vi "IsValidFile.vi"(8 "error in (no error)":errorcluster, 11 "Source Path":path) -> (0 "error out":errorcluster, 2 "Valid File":bool, 3 "path out":path)   [LabVIEW 2023]
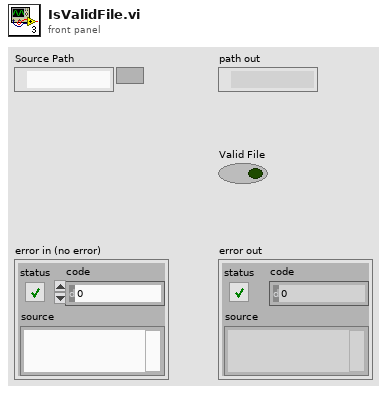
[diagram p1: front panel]
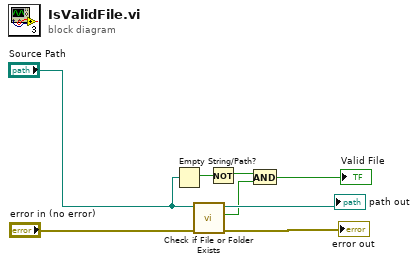
[diagram p0: block diagram]
diagram:
  n1 = Empty String/Path?(string/path="Source Path") -> (empty?=w6:bool)
  n2 = call <vilib>:"Check if File or Folder Exists.vi"("error in (no error)"="error in (no error)", "path"="Source Path") -> ("error out"=→"error out":errorcluster, "file or folder exists?"=w1:bool, "dup path"=→"path out":path)  [unwired: 7 in]
  n3 = Not(x=w6) -> (.not. x?=w7:bool)
  n4 = And(x=w7, y=w1) -> (x .and. y?=→"Valid File":bool)
